vi "Stop Core.vi"(10 "final error code":i32, 11 "FE FF Frame in":refnum<class "FE FF Frame.lvclass">) -> (3 "FE FF Frame out":refnum<class "FE FF Frame.lvclass">)   [LabVIEW 2023, in "Data Analysis.lvlib" / "FE FF Frame.lvlib" / "FE FF Frame.lvclass"]
doc: "(<B>Filename</B>: Actor Framework.lvlib:Actor.lvclass:Stop Core.vi)\n\nDefines what the actor does before it stops. Use the <B>final error code</B> input to determine whether the actor shut down in response to an error.\n\nBy default, this method passes the Stop message along to all auto-stop nested actors. A descendant class may override this method to define additional behavior, such as shutting down any processes the actor initiated in its override of the Actor Core method."
uses:
  FE FF Frame.lvclass
  FE FF Frame.lvclass/FE FF Frame.ctl
  Subpanel-Abstract/Subpanel-Abstract.lvclass
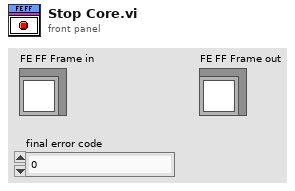
[diagram p1: front panel]
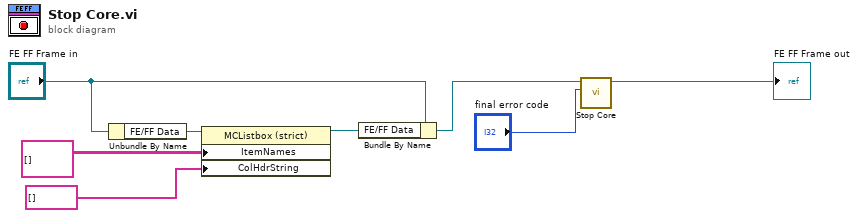
[diagram p0: block diagram]
diagram:
  n1 = Unbundle By Name("FE FF Frame in") -> ("FE/FF Data"=w7:refnum<vi>)
  n2 = property class="MCListbox (strict)"(reference=w7, "ItemNames"=string[][] [] ("Item Names"), "ColHdrString"=string[] [] ("Column Header Strings[]")) -> (reference out=w1:refnum<vi>)  [unwired: 1 in, 1 out]
  n3 = Bundle By Name(cluster="FE FF Frame in", "FE/FF Data"=w1) -> (w2:refnum<class "FE FF Frame.lvclass">)
  n4 = call-parent "Stop Core.vi"("final error code"="final error code", "Actor in"=w2) -> ("Actor out"=→"FE FF Frame out":refnum<class "FE FF Frame.lvclass">)  [unwired: 9 in]
